vi "Car_Speed_R567X.vi"(10 "精度":dbl=1.0, 11 "车速":u16) -> (3 "报文":T1 {"[7]" format="%02x"; "[6]" format="%02x"; "[5]" format="%02x"; "[4]" format="%02x"; "[3]" format="%02x"; "[2]" format="%02x"; "[1]" format="%02x"; "[0]" format="%02x"})   [LabVIEW 2020]
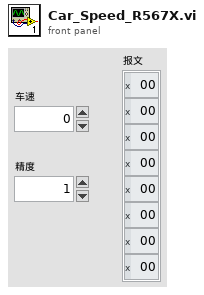
[diagram p1: front panel]
types:
  T1 = cluster{"[0]":u8, "[1]":u8, "[2]":u8, "[3]":u8, "[4]":u8, "[5]":u8, "[6]":u8, "[7]":u8}
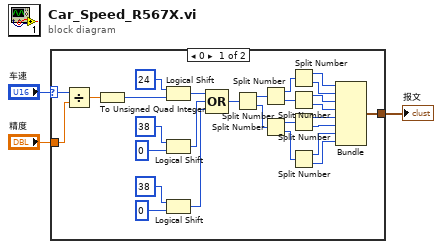
[diagram p0: block diagram]
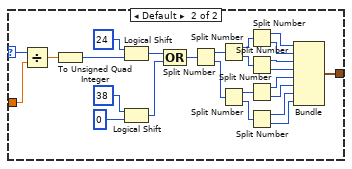
[diagram p2: hidden frame]
diagram:
  n1 = case shown="0" "车速" {
    selector: "车速" -> [w9 w33]
    tunnel: [w7 w40] -> w3
    tunnel: "精度" -> [w8 w32]
    frame 0 {
      n2 = Divide(x=w9, y=w8) -> (x/y=w31:dbl)
      n3 = To Unsigned Quad Integer(1:w31) -> (0:w15:u64)
      n4 = Logical Shift(y=i16 24, x=w15) -> (x << y=w14:u64)
      n5 = Logical Shift(y=i16 38, x=u64 0) -> (x << y=w16:u64)
      n6 = Logical Shift(y=i16 38, x=u64 0) -> (x << y=w4:u64)
      n7 = Compound Arithmetic op=OR ("复合运算")(w14, w16, w4) -> (w13:u64)
      n8 = Split Number(x=w13) -> (hi(x)=w30:u32, lo(x)=w29:u32)
      n9 = Split Number(x=w30) -> (hi(x)=w28:u16, lo(x)=w27:u16)
      n10 = Split Number(x=w29) -> (hi(x)=w26:u16, lo(x)=w25:u16)
      n11 = Split Number(x=w28) -> (hi(x)=w24:u8, lo(x)=w23:u8)
      n12 = Split Number(x=w27) -> (hi(x)=w22:u8, lo(x)=w21:u8)
      n13 = Split Number(x=w26) -> (hi(x)=w20:u8, lo(x)=w19:u8)
      n14 = Split Number(x=w25) -> (hi(x)=w18:u8, lo(x)=w17:u8)
      n15 = Bundle(w24, w23, w22, w21, w20, w19, w18, w17) -> (w7:cluster{u8, u8, u8, u8, u8, u8, u8, u8})  [unwired: 1 in]
    }
    frame Default {
      n16 = Divide(x=w33, y=w32) -> (x/y=w56:dbl)
      n17 = To Unsigned Quad Integer(1:w56) -> (0:w36:u64)
      n18 = Logical Shift(y=i16 24, x=w36) -> (x << y=w35:u64)
      n19 = Logical Shift(y=i16 38, x=u64 0) -> (x << y=w38:u64)
      n20 = Compound Arithmetic op=OR ("复合运算")(w35, w38) -> (w34:u64)
      n21 = Split Number(x=w34) -> (hi(x)=w54:u32, lo(x)=w53:u32)
      n22 = Split Number(x=w54) -> (hi(x)=w52:u16, lo(x)=w51:u16)
      n23 = Split Number(x=w53) -> (hi(x)=w50:u16, lo(x)=w49:u16)
      n24 = Split Number(x=w52) -> (hi(x)=w48:u8, lo(x)=w47:u8)
      n25 = Split Number(x=w51) -> (hi(x)=w46:u8, lo(x)=w45:u8)
      n26 = Split Number(x=w50) -> (hi(x)=w44:u8, lo(x)=w43:u8)
      n27 = Split Number(x=w49) -> (hi(x)=w42:u8, lo(x)=w41:u8)
      n28 = Bundle(w48, w47, w46, w45, w44, w43, w42, w41) -> (w40:cluster{u8, u8, u8, u8, u8, u8, u8, u8})  [unwired: 1 in]
    }
  }
  "报文" <- w3
